vi "example.vi"() -> ()   [LabVIEW 2019]
uses:
  <vilib>/DAQmx/read.llb/DAQmx Read (Analog 1D Wfm NChan NSamp).vi
  <vilib>/DAQmx/create/channels.llb/DAQmx Create Channel (AI-Voltage-Basic).vi
  <vilib>/DAQmx/configure/timing.llb/DAQmx Timing (Sample Clock).vi
  <vilib>/DAQmx/configure/trigger.llb/DAQmx Start Trigger (Analog Edge).vi
  <vilib>/DAQmx/configure/task.llb/DAQmx Configure Logging (TDMS).vi
  <vilib>/DAQmx/miscellaneous.llb/DAQmx Fill In Error Info.vi
  <resource>/objmgr/daqmx.rc
panel:
  out "dt":dbl format="%#.32g"
  out "SampClk.Rate":dbl
  out "Input.OnbrdBufSize":u32
  out "Input.BufSize":u32
  out "Waveform Graph":waveform(dbl)[](graph)
  in  "TDMS File":path
  out "Error Out":errorcluster
  in  "NI-9435":tag
  in  "NI-9775":tag
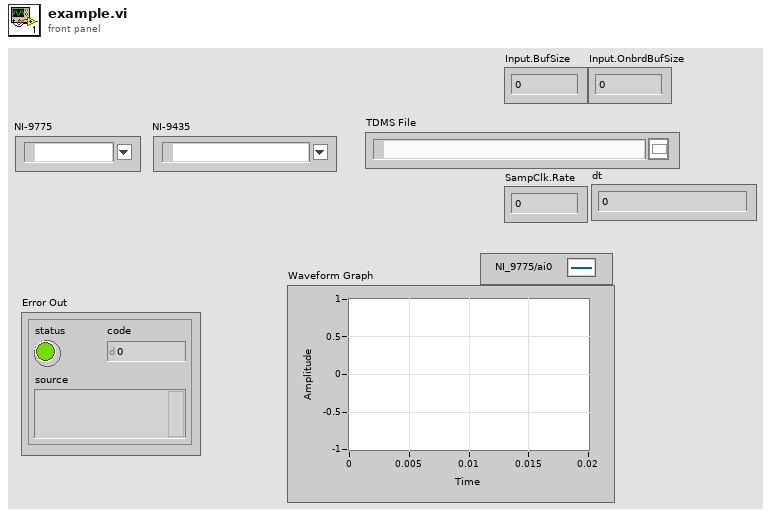
[diagram p1: front panel]
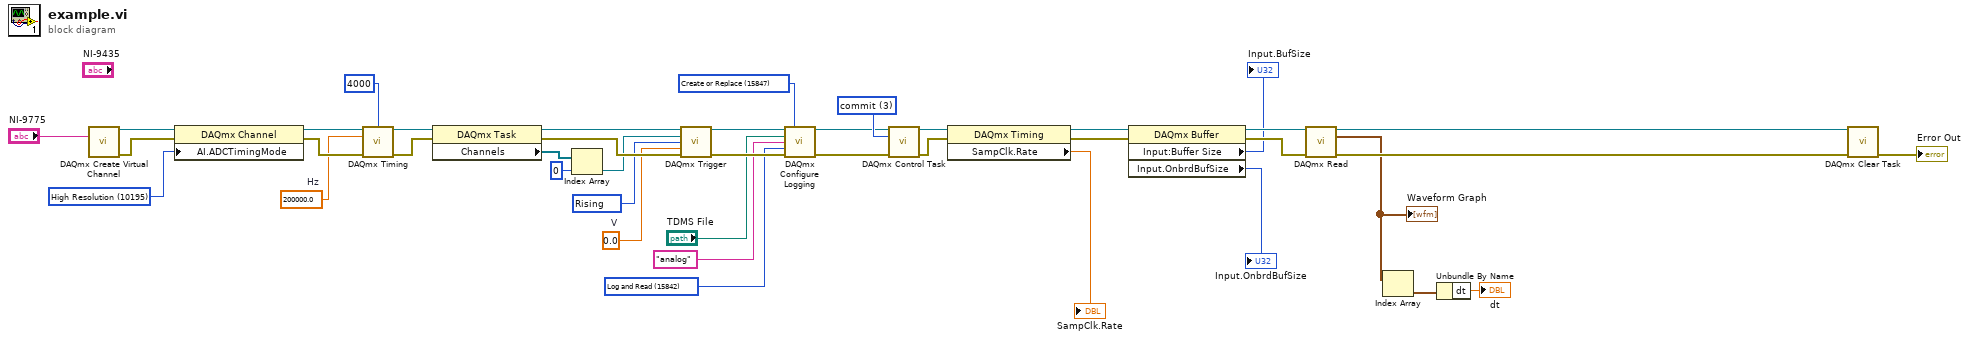
[diagram p0: block diagram]
diagram:
  w11 = 15842 items=["Off"=10231, "Log"=15844, "Log and Read"=15842] ("logging mode")
  w14 = 15847 items=["Open"=10437, "Open or Create"=15846, "Create or Replace"=15847, "Create"=15848] ("operation")
  w27 = 3 items=["verify"=2, "reserve"=4, "commit"=3, "unreserve"=5, "abort"=6] ("action")
  w28 = 0.0  # V
  w29 = 10280 items=["Rising"=10280, "Falling"=10171] ("slope")
  w35 = 200000.0  # Hz
  w38 = 10195 items=["Automatic"=16097, "High Resolution"=10195, "High Speed"=14712, "Best 50 Hz Rejection"=14713, "Best 60 Hz Rejection"=14714, "Custom"=10137] ("AI.ADCTimingMode")
  n1 = call-poly <vilib>:"DAQmx Create Virtual Channel.vi"("physical channels"="NI-9775") -> ("task out"=w40:refnum<k21>, "error out"=w39:errorcluster)  [unwired: 13 in]
  n2 = property class="DAQmx Channel"(reference=w40, error in=w39, "AI.ADCTimingMode"=w38) -> (reference out=w37:refnum<k21>, error out=w36:errorcluster)
  n3 = call-poly <vilib>:"DAQmx Timing.vi"("task/channels in"=w37, "samples per channel"=4000, "rate"=w35, "error in"=w36) -> ("task out"=w24:refnum<k21>, "error out"=w25:errorcluster)  [unwired: 10 in]
  n4 = property class="DAQmx Task"(reference=w24, error in=w25) -> (reference out=w31:refnum<k21>, error out=w32:errorcluster, "Channels"=w34:refnum<k21>[])
  n5 = Index Array(array=w34, index=0) -> (element=w30:refnum<k21>)
  n6 = call-poly <vilib>:"DAQmx Trigger.vi"("task/channels in"=w31, "source"=w30, "slope"=w29, "level"=w28, "error in"=w32) -> ("task out"=w15:refnum<k21>, "error out"=w16:errorcluster)  [unwired: 9 in]
  n7 = call-poly <vilib>:"DAQmx Configure Logging.vi"("task/channels in"=w15, "operation"=w14, "file path"="TDMS File", "group name"="analog", "logging mode"=w11, "error in"=w16) -> ("task out"=w9:refnum<k21>, "error out"=w10:errorcluster)  [unwired: 8 in]
  n8 = call <vilib>:"DAQmx Control Task.vi"("task/channels in"=w9, "action"=w27, "error in"=w10) -> ("task out"=w8:refnum<k21>, "error out"=w7:errorcluster)  [unwired: 11 in]
  n9 = property class="DAQmx Timing"(reference=w8, error in=w7) -> (reference out=w5:refnum<k21>, error out=w6:errorcluster, "SampClk.Rate"=→"SampClk.Rate":dbl)
  n10 = property class="DAQmx Buffer"(reference=w5, error in=w6) -> (reference out=w20:refnum<k21>, error out=w19:errorcluster, "Input:Buffer Size"=→"Input.BufSize":u32, "Input.OnbrdBufSize"=→"Input.OnbrdBufSize":u32)
  n11 = call-poly <vilib>:"DAQmx Read.vi"("task/channels in"=w20, "error in"=w19) -> ("task out"=w22:refnum<k21>, "data"=w3:waveform(dbl)[], "error out"=w23:errorcluster)  [unwired: 11 in]
  "Waveform Graph" <- w3
  n12 = Index Array(array=w3) -> (element=w2:waveform(dbl))  [unwired: 1 in]
  n13 = Unbundle By Name(w2) -> ("dt"=→"dt":dbl)
  n14 = call <vilib>:"DAQmx Clear Task.vi"("task in"=w22, "error in"=w23) -> ("error out"=→"Error Out":errorcluster)  [unwired: 13 in]
